vi "XML File Version Migration.vi"() -> ()   [LabVIEW 2011, in "XML VIs.lvlib"]
uses:
  XML VIs.lvlib
panel:
  out "error out":errorcluster
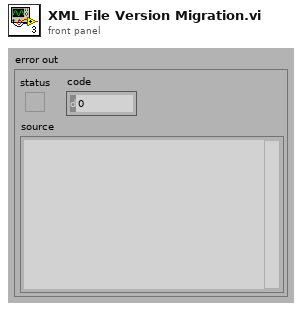
[diagram p1: front panel]
types:
  T1 = typedef "Type Definitions.lvlib/Type FOFB Parameters.ctl" = cluster{"Network":T2, "Fast Acquisition":T3, "Response Matrix Measurement":T4, "Correction Algorithm":T5, "Acquisition Network":T6, "Actuation Network":T7}
  T2 = typedef "Type Definitions.lvlib/Type Network Configuration.ctl" = cluster{"FOFB Controller IP":string, "LNLS Control Network IP":string, "LNLS Control Network Power Supplies TCP Port":u16, "LNLS Control Network FOFB Configuration TCP Port":u16, "MML Data Server TCP Port":u16, "Monitoring Data TCP Port":u16, "Configuration GUI TCP Port":u16, "TCP Listening Timeout":i32}
  T3 = typedef "Type Definitions.lvlib/Type FA Configuration.ctl" = cluster{"Acquisition Period":u32, "Data Buffer Size":u32}
  T4 = typedef "Type Definitions.lvlib/Type Response Matrix Measurement Configuration.ctl" = cluster{"Step Amplitude":dbl, "Time Between Steps":u32, "Step Duration":u32, "Number of Averages":u32}
  T5 = typedef "Type Definitions.lvlib/Type Correction Algorithm Configuration.ctl" = cluster{"Correction Period":u32, "Reference Orbit Path":path, "Response Matrix Path":path, "Correction Matrix Path":path, "Horizontal Correction Factor":dbl, "Vertical Correction Factor":dbl, "Beam Current FOFB Threshold":dbl, "Decouple H-V":bool}
  T6 = typedef "Type Definitions.lvlib/Type Acquisition Network Configuration.ctl" = cluster{"Chassis Name":string, "Variables":cluster{"Variable Name":string, "Matrix Order":u32, "Location":dbl, "Plane":enum8{"H", "V"}, "On Correction":bool}[]}[]
  T7 = typedef "Type Definitions.lvlib/Type Actuation Network Configuration.ctl" = cluster{"Chassis Name":string, "Variables":cluster{"Variable Name":string, "Matrix Order":u32, "RMM Step Factor":dbl, "Plane":enum8{"H", "V"}, "On Correction":bool, "Kc":dbl, "Ti":dbl, "Td":dbl}[]}[]
  T8 = cluster{"FOFB Controller IP":string, "LNLS Control Network IP":string, "LNLS Control Network Power Supplies TCP Port":u16, "LNLS Control Network FOFB Configuration TCP Port":u16, "MML Data Server TCP Port":u16, "Monitoring Data TCP Port":u16, "Configuration GUI TCP Port":u16, "TCP Listening Timeout":i32}
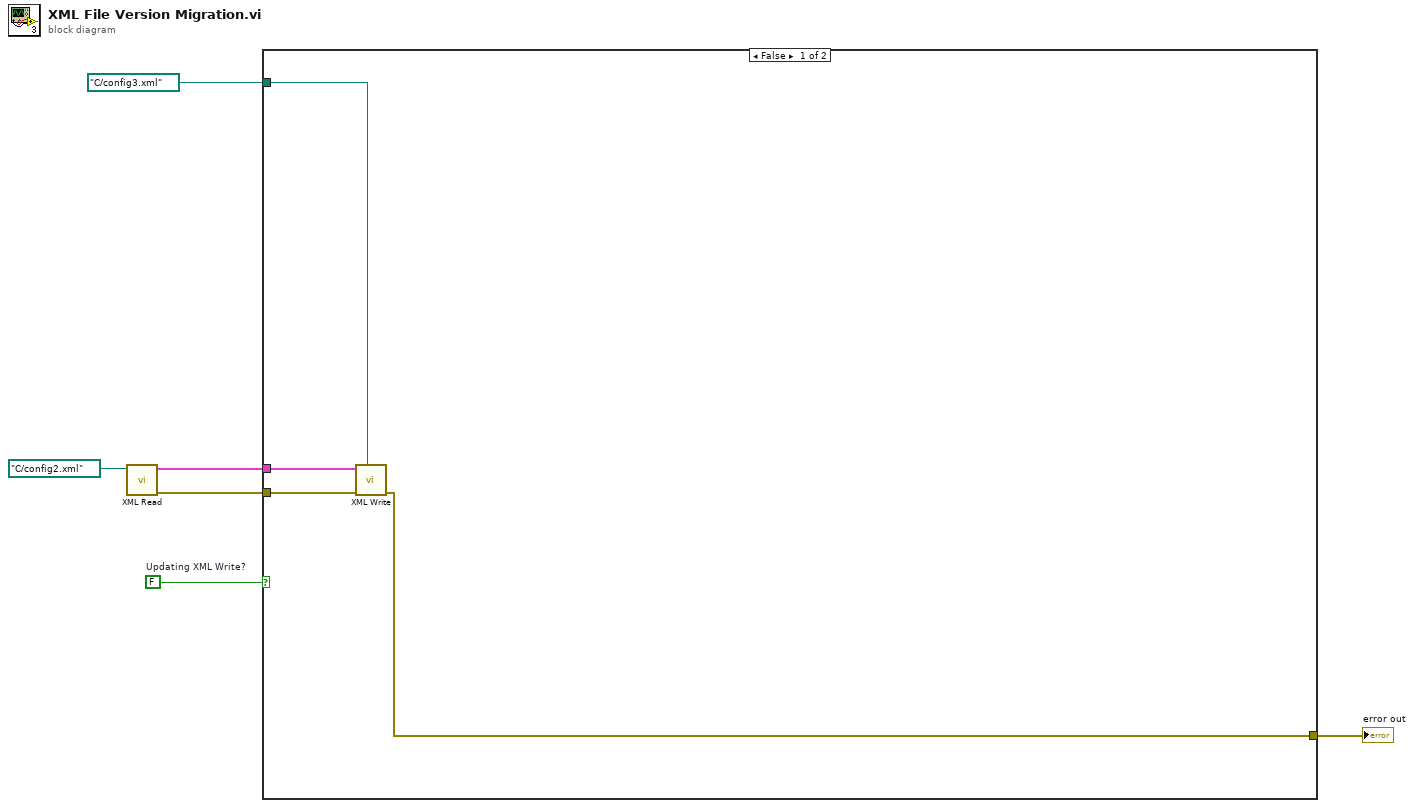
[diagram p0: block diagram]
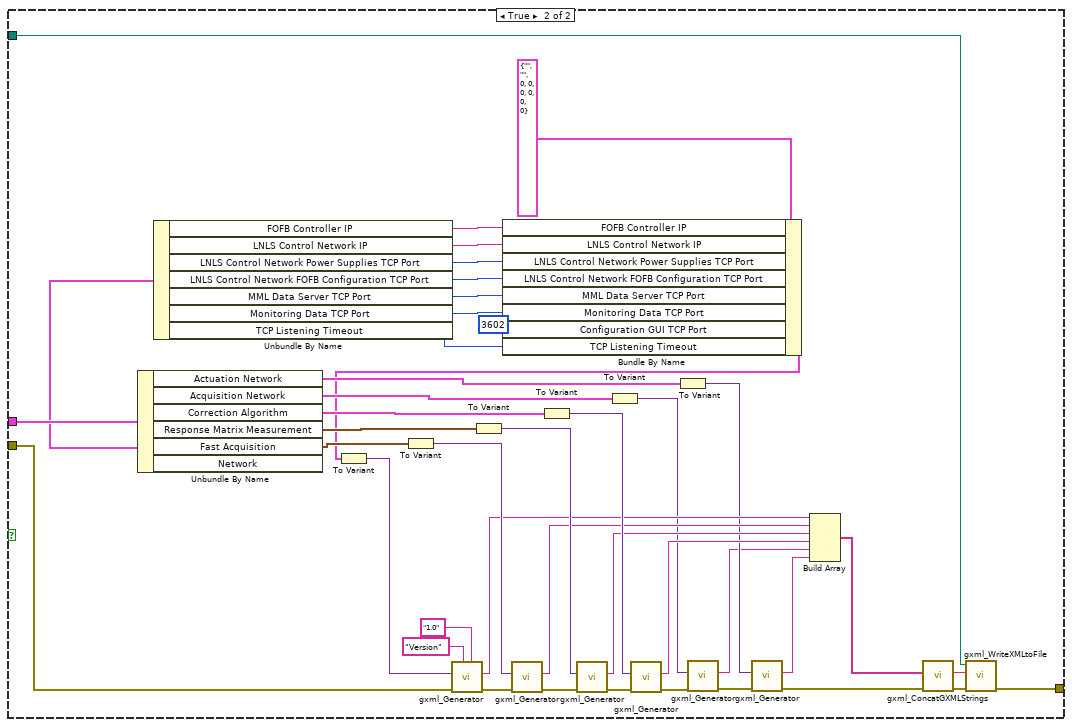
[diagram p2: hidden frame]
diagram:
  w1 = FALSE  # Updating XML Write?
  n1 = call "XML Read.vi"("XML File Path In"=path "C:/config2.xml") -> ("error out"=w4:errorcluster, "FOFB Parameters"=w5:T1)  [unwired: 9 in]
  n2 = case shown="False" w1 {
    tunnel: [w9 w27] -> w6
    tunnel: w5 -> [w8 w26]
    tunnel: w4 -> [w10 w25]
    tunnel: path "C:/config3.xml" ("XML File Path In") -> [w7 w24]
    frame False {
      n3 = call "XML Write.vi"("XML File Path Write"=w7, "Error In"=w10, "FOFB Parameters"=w8) -> ("Error Out"=w9:errorcluster)  [unwired: 7 in, 1 out]
    }
    frame True {
      n4 = Unbundle By Name(w26) -> ("Actuation Network"=w22:T7, "Acquisition Network"=w28:T6, "Correction Algorithm"=w23:T5, "Response Matrix Measurement"=w29:T4, "Fast Acquisition"=w30:T3, "Network"=w21:T2)
      n5 = Unbundle By Name(w21) -> ("FOFB Controller IP"=w20:string, "LNLS Control Network IP"=w19:string, "LNLS Control Network Power Supplies TCP Port"=w17:u16, "LNLS Control Network FOFB Configuration TCP Port"=w16:u16, "MML Data Server TCP Port"=w15:u16, "Monitoring Data TCP Port"=w14:u16, "TCP Listening Timeout"=w13:i32)
      n6 = To Variant(anything=w30) -> (Variant=w40:variant)
      n7 = To Variant(anything=w29) -> (Variant=w44:variant)
      n8 = Bundle By Name(cluster=T8 {"FOFB Controller IP"="", "LNLS Control Network IP"="", "LNLS Control Network Power Supplies TCP Port"=0, "LNLS Control Network FOFB Configuration TCP Port"=0, "MML Data Server TCP Port"=0, "Monitoring Data TCP Port"=0, "Configuration GUI TCP Port"=0, "TCP Listening Timeout"=0} ("Network"), "FOFB Controller IP"=w20, "LNLS Control Network IP"=w19, "LNLS Control Network Power Supplies TCP Port"=w17, "LNLS Control Network FOFB Configuration TCP Port"=w16, "MML Data Server TCP Port"=w15, "Monitoring Data TCP Port"=w14, "Configuration GUI TCP Port"=u16 3602, "TCP Listening Timeout"=w13) -> (w11:T8)
      n9 = To Variant(anything=w11) -> (Variant=w41:variant)
      n10 = call "gxml_Generator.vi"("Version String"="1.0", "Version Tag Name"="Version", "error in"=w25, "Variant"=w41) -> ("error out"=w42:errorcluster, "XML String Out"=w38:string)  [unwired: 6 in]
      n11 = call "gxml_Generator.vi"("error in"=w42, "Variant"=w40) -> ("error out"=w45:errorcluster, "XML String Out"=w39:string)  [unwired: 8 in]
      n12 = To Variant(anything=w23) -> (Variant=w48:variant)
      n13 = call "gxml_Generator.vi"("error in"=w45, "Variant"=w44) -> ("error out"=w43:errorcluster, "XML String Out"=w46:string)  [unwired: 8 in]
      n14 = To Variant(anything=w28) -> (Variant=w35:variant)
      n15 = call "gxml_Generator.vi"("error in"=w43, "Variant"=w48) -> ("error out"=w33:errorcluster, "XML String Out"=w47:string)  [unwired: 8 in]
      n16 = To Variant(anything=w22) -> (Variant=w34:variant)
      n17 = call "gxml_Generator.vi"("error in"=w33, "Variant"=w35) -> ("error out"=w37:errorcluster, "XML String Out"=w32:string)  [unwired: 8 in]
      n18 = call "gxml_Generator.vi"("error in"=w37, "Variant"=w34) -> ("error out"=w36:errorcluster, "XML String Out"=w31:string)  [unwired: 8 in]
      n19 = Build Array(w38, w39, w46, w47, w32, w31) -> (w51:string[])
      n20 = call "gxml_ConcatGXMLStrings.vi"("error in"=w36, "GXML Strings"=w51) -> ("error out"=w52:errorcluster, "Concatenated GXML String"=w53:string)  [unwired: 8 in]
      n21 = call "gxml_WriteXMLtoFile.vi"("error in"=w52, "XML Input"=w53, "XML File Path"=w24) -> ("error out"=w27:errorcluster)  [unwired: 7 in, 1 out]
    }
  }
  "error out" <- w6
